vi "625CubeLaser.vi"() -> ()   [LabVIEW 2011]
panel:
  out "625Cube":bool
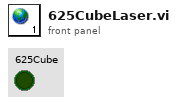
[diagram p1: front panel]
diagram:
